vi "Character Maker.vi"() -> ()   [LabVIEW 2010]
doc: "This program is used to design characters and then generate the corresponding key-value pairs to enter into the configuration file under a corresponding section. So, when the user requests a given character to be scrolled across the Moving Message Board display, the corresponding key-value pairs will be read from the configuration file and processed to produce the scrolling letter. The program has the ability to load the key-value pairs from an existing character (a section in the configuration file), and then display the corresponding character in the Character array. At this point, the Character array can be modified and a new set of key-value pairs can be generated, if desired. Of course the Character array can be used to make any design, not just the characters from the keyboard. The user could, for example make a picture of a fish in the Character array and map that to the letter \"A\"."
uses:
  Instance           1 33Saved   Character Maker With Load .vi
  <vilib>/Utility/config.llb/Read Key (I32).vi
  <vilib>/Utility/config.llb/NI_LVConfig.lvlib
panel:
  in  "Config Path":path=path "c:/Ed's Files/LabVIEW Files/Moving Message Board/mmb.ini"
  in  "Load Config":bool
  in  "Clear":bool
  in  "stop":bool
  in  "Make Config":bool
  out "String":string
  in  "Character":bool[][](array[boolean])
  # "9"
  # "9"
  # "9"
  # "9"
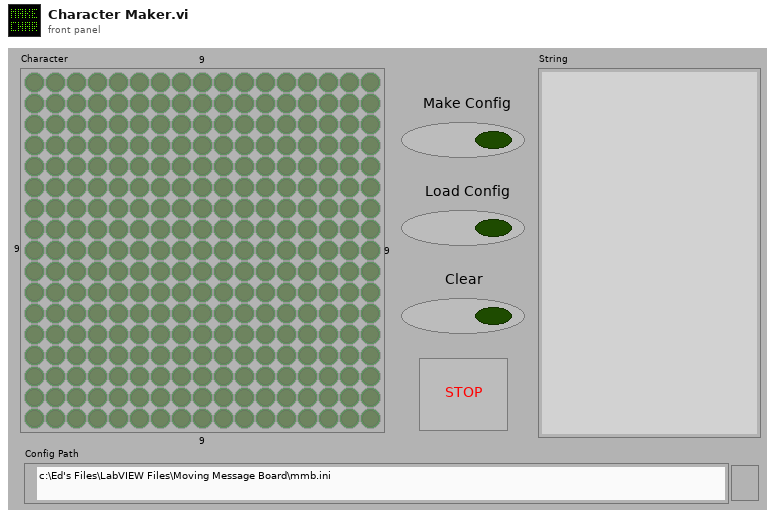
[diagram p1: front panel]
types:
  T1 = typedef "NI_LVConfig.lvlib/Config Data RefNum.ctl" = refnum<k1>
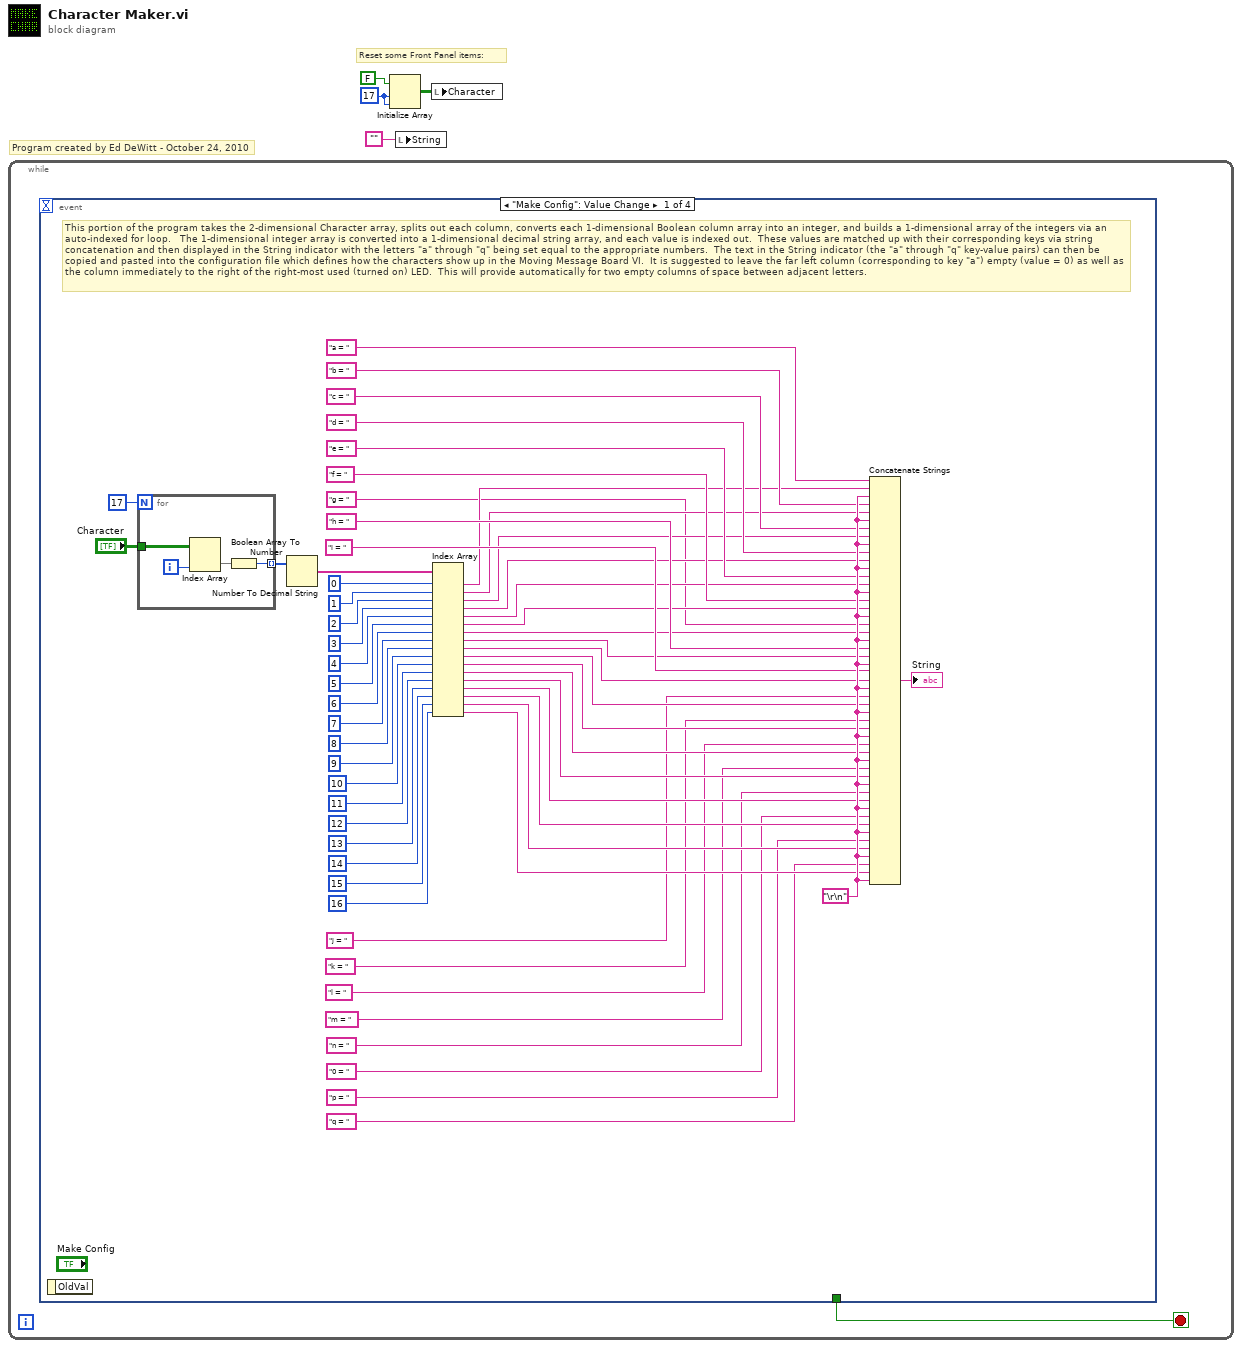
[diagram p0: block diagram]
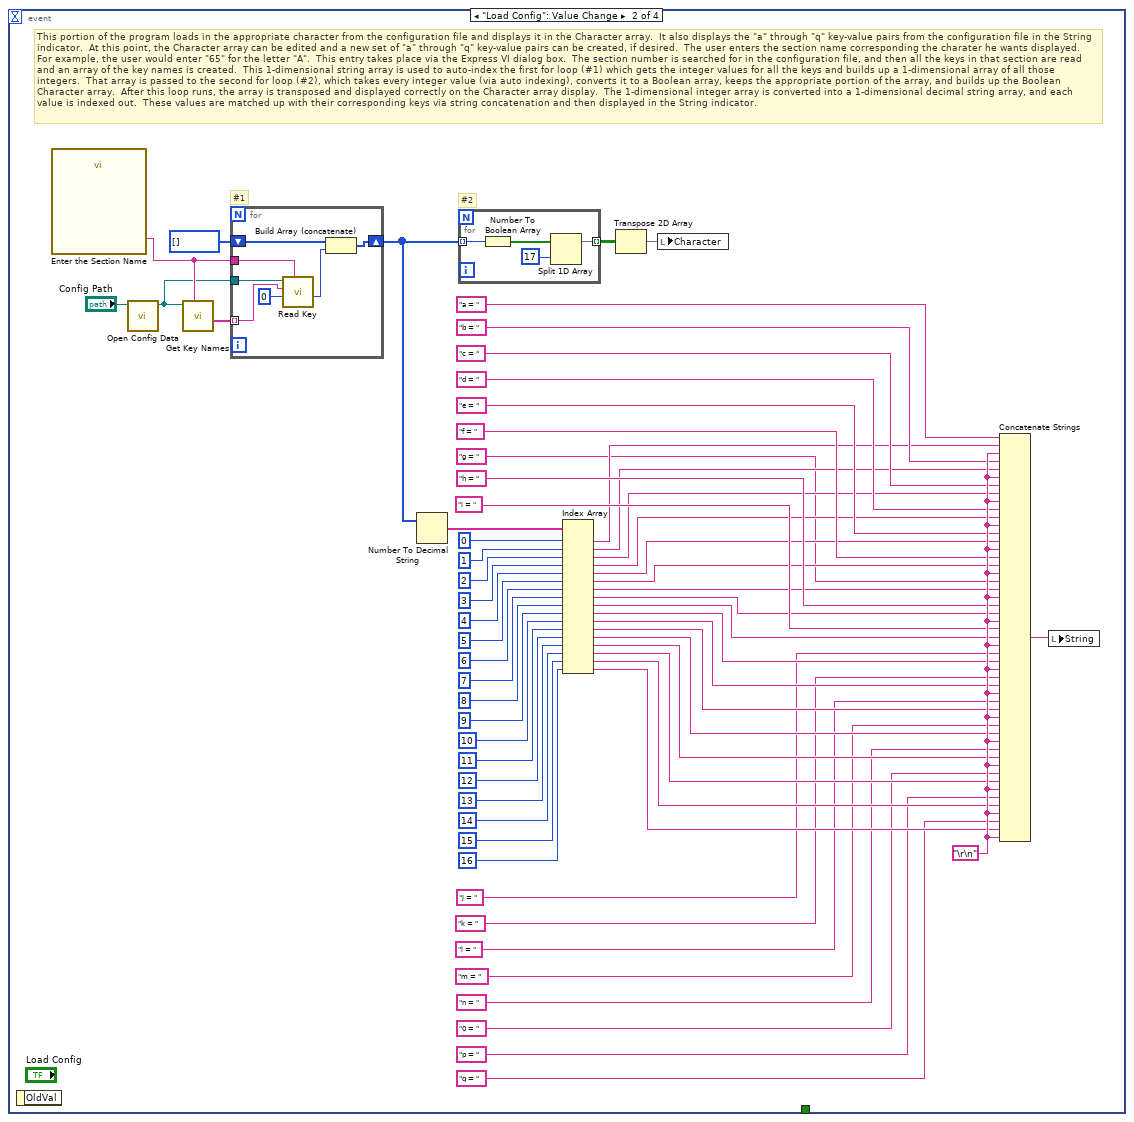
[diagram p2: hidden frame]
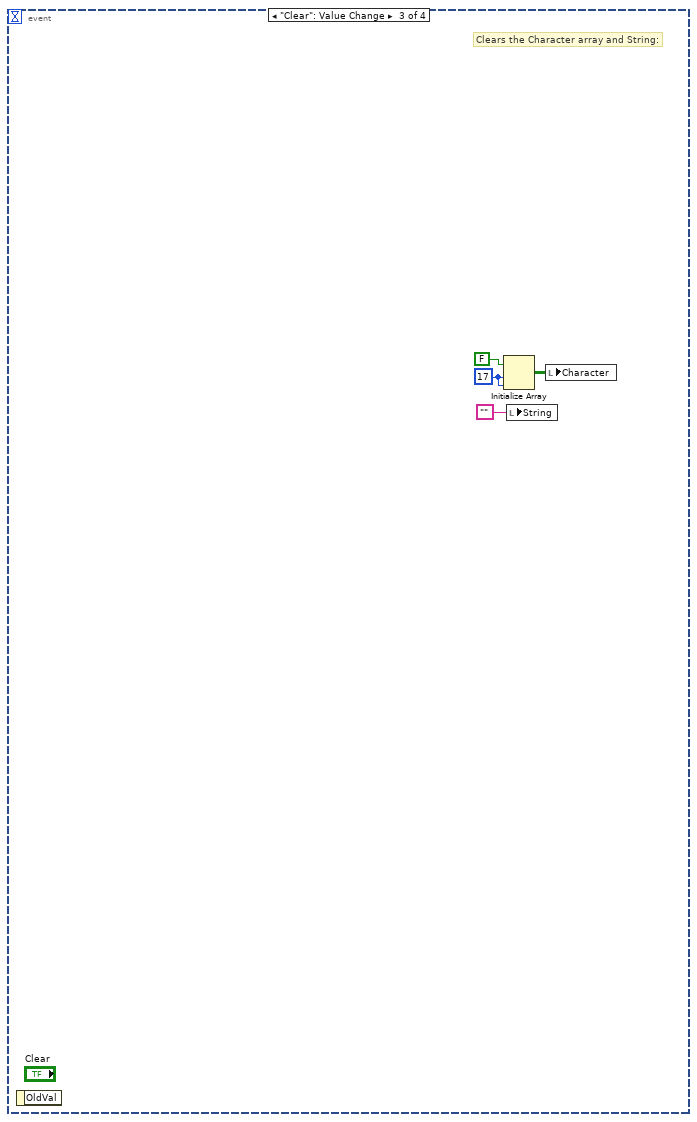
[diagram p3: hidden frame]
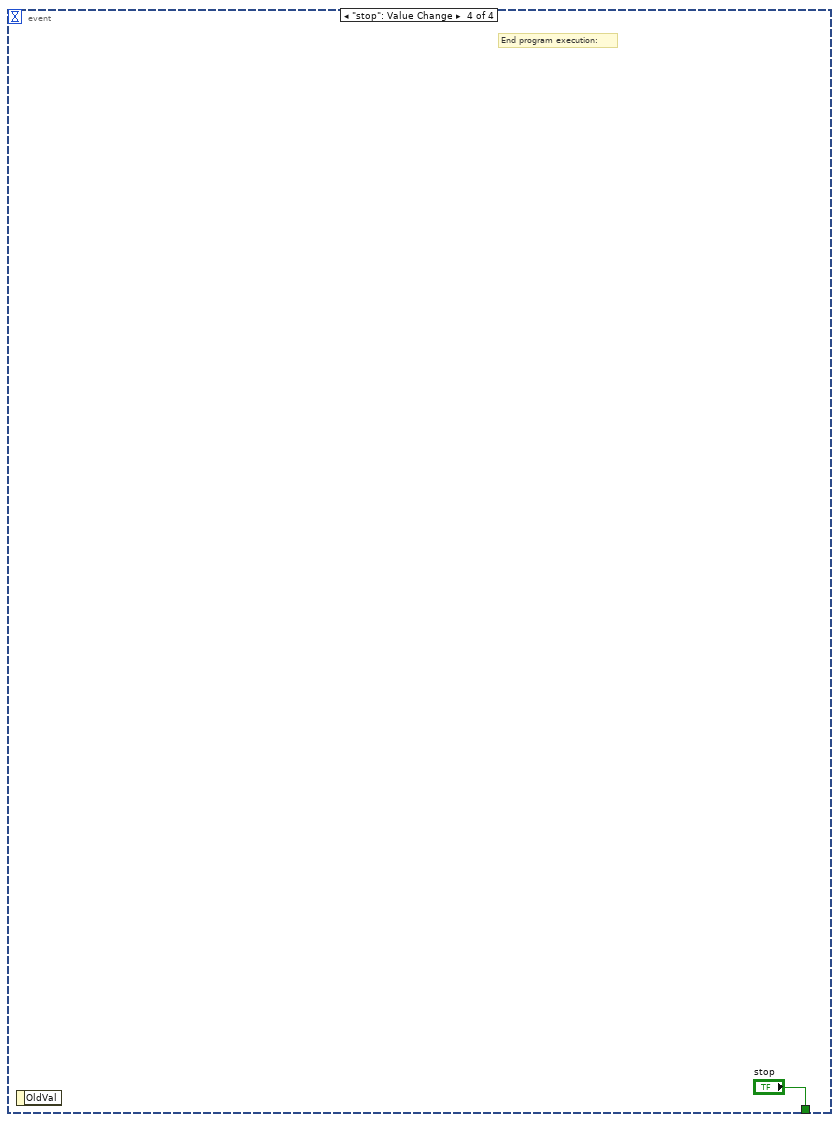
[diagram p4: hidden frame]
diagram:
  w3 = 17 ("dimension size")
  # "Program created by Ed DeWitt - October 24, 2010"
  # "Reset some Front Panel items:"
  n1 = while {
    stop <- w5 stop-if-true
    n2 = event shown="[0] \"Make Config\": Value Change" {
      selector: _ -> [_ _ _ _]
      dyn-events: _ -> [_ _ _ _]
      timeout: _ -> [_ _ _ _]
      tunnel: [_ _ _ "stop"] -> w5
      event "Make Config": Value Change {
        w61 = "\r\n"
        # "This portion of the program takes the 2-dimensional Character array, splits out each column, converts each 1-dimensional Boolean column array into an integer, and builds a 1-dimensional array of the integers via an auto-indexed for loop.   The 1-dimensional integer array is converted into a 1-dimensional decimal string array, and each value is indexed out.  These values are matched up with their corresponding keys via string concatenation and then displayed in the String indicator with the letters \"a\" through \"q\" being set equal to the appropriate numbers.  The text in the String indicator (the \"a\" through \"q\" key-value pairs) can then be copied and pasted into the configuration file which defines how the characters show up in the Moving Message Board VI.  It is suggested to leave the far left column (corresponding to key \"a\") empty (value = 0) as well as the column immediately to the right of the right-most used (turned on) LED.  This will provide automatically for two empty columns of space between adjacent letters."
        n3 = event-data() -> ()  [unwired: 1 in, 1 out]
        n4 = for {
          N: 17 -> [_]
          tunnel: "Character" -> [w66]
          tunnel: [w63] -> w27 mode=indexing
          i -> [w65]
          n5 = Index Array(array=w66, index (col)=w65) -> (element=w64:bool[])  [unwired: 1 in]
          n6 = Boolean Array To Number(Boolean array=w64) -> (number=w63:u32)
        }
        n7 = Number To Decimal String(number=w27) -> (decimal integer string=w28:string[])  [unwired: 1 in]
        n8 = Index Array(array=w28, index #1=0 ("index"), index #2=1 ("index"), index #3=2 ("index"), index #4=3 ("index"), index #5=4 ("index"), index #6=5 ("index"), index #7=6 ("index"), index #8=7 ("index"), index #9=8 ("index"), index #10=9 ("index"), index #11=10 ("index"), index #12=11 ("index"), index #13=12 ("index"), index #14=13 ("index"), index #15=14 ("index"), index #16=15 ("index"), index #17=16 ("index")) -> (element #1=w30:string, element #2=w7:string, element #3=w33:string, element #4=w35:string, element #5=w37:string, element #6=w39:string, element #7=w40:string, element #8=w42:string, element #9=w44:string, element #10=w46:string, element #11=w48:string, element #12=w50:string, element #13=w52:string, element #14=w54:string, element #15=w56:string, element #16=w59:string, element #17=w60:string)
        n9 = Concatenate Strings("a = ", w30, w61, "b = ", w7, w61, "c = ", w33, w61, "d = ", w35, w61, "e = ", w37, w61, "f = ", w39, w61, "g = ", w40, w61, "h = ", w42, w61, "i = ", w44, w61, "j = ", w46, w61, "k = ", w48, w61, "l = ", w50, w61, "m = ", w52, w61, "n = ", w54, w61, "0 = ", w56, w61, "p = ", w59, w61, "q = ", w60, w61) -> (→"String":string)
      }
      event "Load Config": Value Change {
        w126 = "\r\n"
        # "#2"
        # "#1"
        # "This portion of the program loads in the appropriate character from the configuration file and displays it in the Character array.  It also displays the \"a\" through \"q\" key-value pairs from the configuration file in the String indicator.  At this point, the Character array can be edited and a new set of \"a\" through \"q\" key-value pairs can be created, if desired.  The user enters the section name corresponding the charater he wants displayed.  For example, the user would enter \"65\" for the letter \"A\".  This entry takes place via the Express VI dialog box.  The section number is searched for in the configuration file, and then all the keys in that section are read and an array of the key names is created.  This 1-dimensional string array is used to auto-index the first for loop (#1) which gets the integer values for all the keys and builds up a 1-dimensional array of all those integers.  That array is passed to the second for loop (#2), which takes every integer value (via auto indexing), converts it to a Boolean array, keeps the appropriate portion of the array, and builds up the Boolean Character array.  After this loop runs, the array is transposed and displayed correctly on the Character array display.  The 1-dimensional integer array is converted into a 1-dimensional decimal string array, and each value is indexed out.  These values are matched up with their corresponding keys via string concatenation and then displayed in the String indicator."
        n10 = event-data() -> ()  [unwired: 1 in, 1 out]
        n11 = call "Enter the Section Name"() -> ("Section"=w70:string)  [unwired: 17 in, 2 out]
        n12 = call <vilib>:"Open Config Data.vi"("configuration file path"="Config Path") -> ("refnum"=w68:T1)  [unwired: 8 in, 2 out]
        n13 = call <vilib>:"Get Key Names.vi"("section"=w70, "refnum"=w68) -> ("key names"=w71:string[])  [unwired: 6 in, 3 out]
        n14 = for {
          tunnel: w71 -> [w134] mode=indexing
          tunnel: w68 -> [w133]
          shift-right: [w129] -> w73
          shift-left: i32[] [] -> [w130]
          tunnel: w70 -> [w135]
          n15 = call-poly <vilib>:"Read Key.vi"("section"=w135, "default value"=0, "key"=w134, "refnum"=w133) -> ("value"=w132:i32)  [unwired: 4 in, 3 out]
          n16 = Build Array (concatenate)(w130, w132) -> (w129:i32[])
        }
        n17 = Number To Decimal String(number=w73) -> (decimal integer string=w93:string[])  [unwired: 1 in]
        n18 = for {
          tunnel: w73 -> [w137] mode=indexing
          tunnel: [w136] -> w128 mode=indexing
          n19 = Number To Boolean Array(number=w137) -> (Boolean array=w139:bool[])
          n20 = Split 1D Array(array=w139, index=17) -> (first subarray=w136:bool[])  [unwired: 1 out]
        }
        n21 = Index Array(array=w93, index #1=0 ("index"), index #2=1 ("index"), index #3=2 ("index"), index #4=3 ("index"), index #5=4 ("index"), index #6=5 ("index"), index #7=6 ("index"), index #8=7 ("index"), index #9=8 ("index"), index #10=9 ("index"), index #11=10 ("index"), index #12=11 ("index"), index #13=12 ("index"), index #14=13 ("index"), index #15=14 ("index"), index #16=15 ("index"), index #17=16 ("index")) -> (element #1=w95:string, element #2=w75:string, element #3=w98:string, element #4=w100:string, element #5=w102:string, element #6=w104:string, element #7=w105:string, element #8=w107:string, element #9=w109:string, element #10=w111:string, element #11=w113:string, element #12=w115:string, element #13=w117:string, element #14=w119:string, element #15=w121:string, element #16=w124:string, element #17=w125:string)
        n22 = Transpose 2D Array(2D array=w128) -> (transposed array=w127:bool[][])
        n23 = local write "Character"(w127) -> ()
        n24 = Concatenate Strings("a = ", w95, w126, "b = ", w75, w126, "c = ", w98, w126, "d = ", w100, w126, "e = ", w102, w126, "f = ", w104, w126, "g = ", w105, w126, "h = ", w107, w126, "i = ", w109, w126, "j = ", w111, w126, "k = ", w113, w126, "l = ", w115, w126, "m = ", w117, w126, "n = ", w119, w126, "0 = ", w121, w126, "p = ", w124, w126, "q = ", w125, w126) -> (w72:string)
        n25 = local write "String"(w72) -> ()
      }
      event "Clear": Value Change {
        w142 = 17 ("dimension size")
        # "Clears the Character array and String:"
        n26 = event-data() -> ()  [unwired: 1 in, 1 out]
        n27 = Initialize Array(FALSE, w142, w142) -> (w141:bool[][])
        n28 = local write "String"("") -> ()
        n29 = local write "Character"(w141) -> ()
      }
      event "stop": Value Change {
        # "End program execution:"
        n30 = event-data() -> ()  [unwired: 1 in, 1 out]
      }
    }
  }
  n31 = Initialize Array(FALSE, w3, w3) -> (w4:bool[][])
  n32 = local write "String"("") -> ()
  n33 = local write "Character"(w4) -> ()
